vi "Delete All Modbus Channels.vi"(8 "error in (no error)":errorcluster, 11 "CD Ref In":T1 format="%.0x") -> (0 "error out":errorcluster)   [LabVIEW 2014, in "Modbus System Explorer.lvlib"]
uses:
  Modbus System Explorer.lvlib
  <vilib>/NI Veristand/Custom Device API/Custom Device Item Ref.ctl
  Shared/Modbus GUID Lookup.vi
  <vilib>/NI Veristand/Custom Device Tools/Custom Device Utility Library/NI VeriStand - Search for All Items by GUID.vi
  <vilib>/NI Veristand/Custom Device Tools/Custom Device Utility Library/Custom Device Utility Library.lvlib
  Shared/Modbus Shared.lvlib
  <vilib>/NI Veristand/Custom Device API/Custom Device API.lvlib
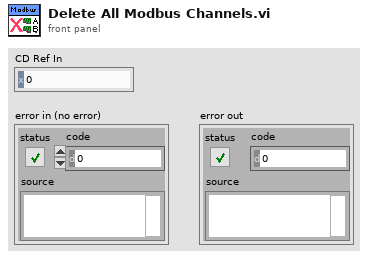
[diagram p1: front panel]
types:
  T1 = typedef "Custom Device API.lvlib/Custom Device Item Ref.ctl" = u64
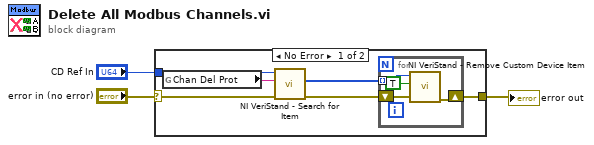
[diagram p0: block diagram]
diagram:
  n1 = case shown="No Error" "error in (no error)" {
    selector: "error in (no error)" -> [w4 w14]
    tunnel: "CD Ref In" -> [w6 _]
    tunnel: [w5 w14] -> w2
    frame No Error {
      n2 = global read "Modbus GUID Lookup.vi" "Chan Del Prot"() -> (w9:string)
      n3 = call-poly <vilib>:"NI VeriStand - Search for Item.vi"("error in"=w4, "Item GUID"=w9, "Section Ref in"=w6) -> ("error out"=w8:errorcluster, "Item Refs"=w7:T1[])  [unwired: 5 in, 2 out]
      n4 = for {
        shift-right: [w12] -> w5
        shift-left: w8 -> [w13]
        tunnel: w7 -> [w11] mode=indexing
        n5 = call <vilib>:"NI VeriStand - Remove Custom Device Item.vi"("error in (no error)"=w13, "Force Delete (F)"=TRUE, "Item Ref in"=w11) -> ("error out"=w12:errorcluster)  [unwired: 7 in, 1 out]
      }
    }
    frame Error {
    }
  }
  "error out" <- w2
